vi "Read Configuration File.vi"(0 "Device Type":T1=enum."Stage", 11 "Device Function":T2=enum."Secondary", 13 "Config File Path":path) -> (2 "Configuration Name":string, 4 "Unique Notifier Name":string, 8 "Device Ports/IDs/Channels":string[](array[string]), 15 "Device Engine Path":path)   [LabVIEW 2016]
uses:
  Hardware Configuration Controls/Device Function.ctl
  Hardware Configuration Controls/Device Type.ctl
panel:
  out "File Lines":string[](array[string])
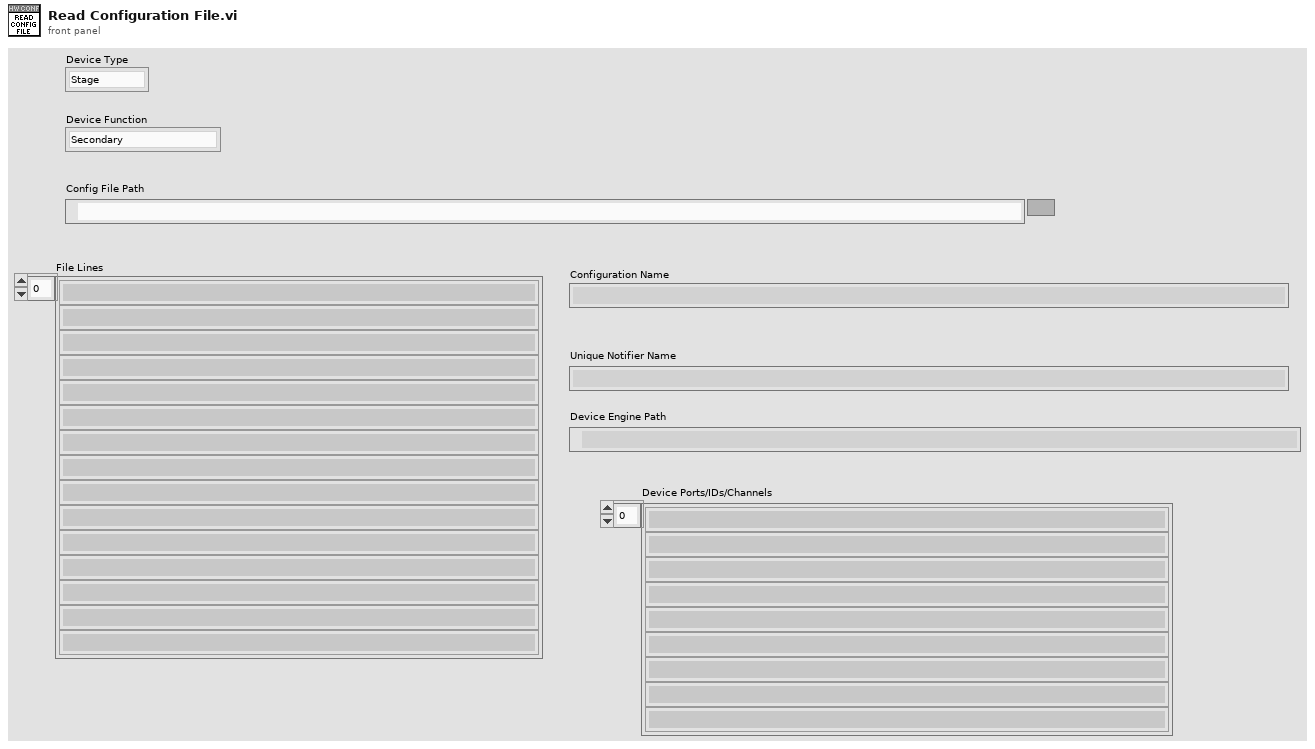
[diagram p1: front panel]
types:
  T1 = typedef "Device Type.ctl" = enum16{"AOTF", "Camera", "Deformable Mirror", "Laser", "Shutter", "Stage", "Waveform", "Email"}
  T2 = typedef "Device Function.ctl" = enum16{"Primary", "Secondary", "Overview", "Wide Field Drift Correction", "642 nm Excitation", "560 nm Excitation", "546 nm Excitation", "488 nm Excitation", "405 nm Excitation", "Objective Drift Correction", "Objective XY", "Objective Z", "Sample XY", "Sample Coarse Z", "Sample Z", "4Pi Lower", "4Pi Upper", "Adj Cavity", "Line Scanning", "Alert"}
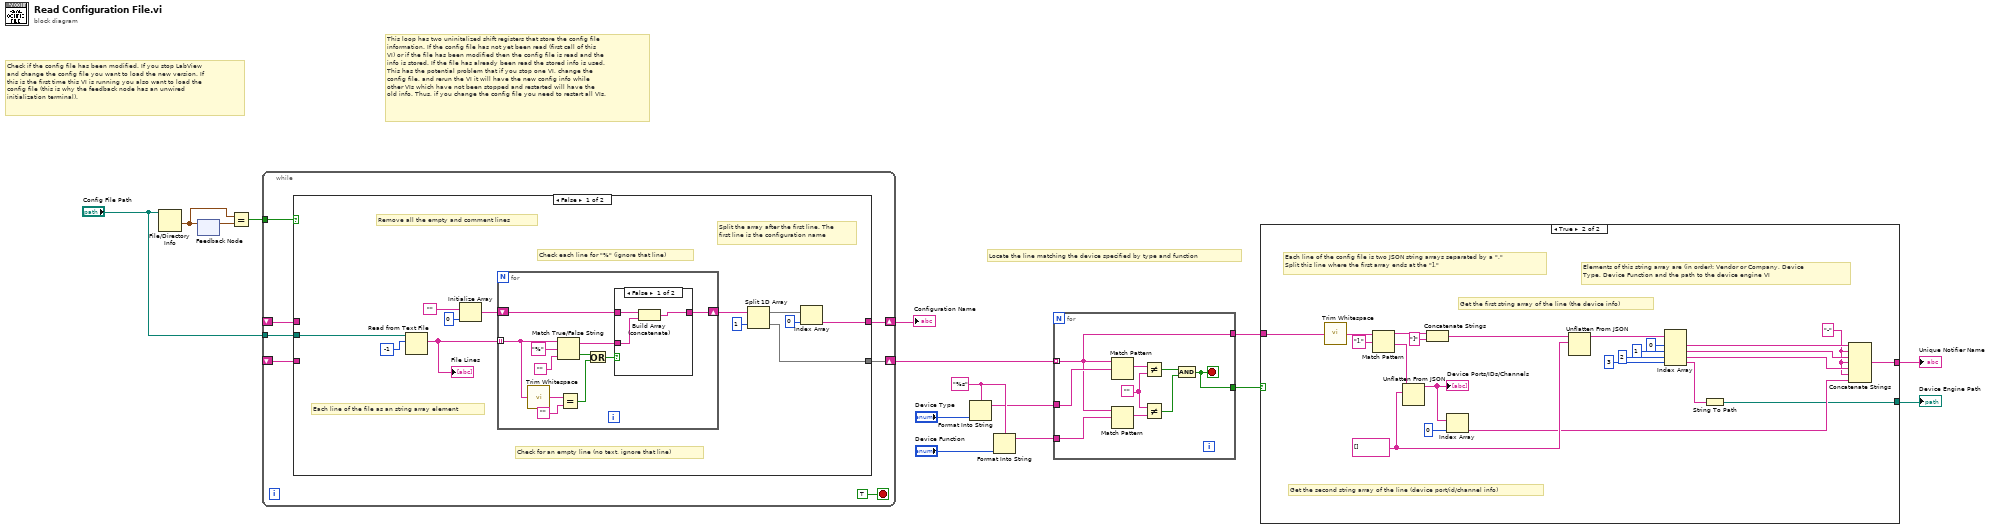
[diagram p0: block diagram]
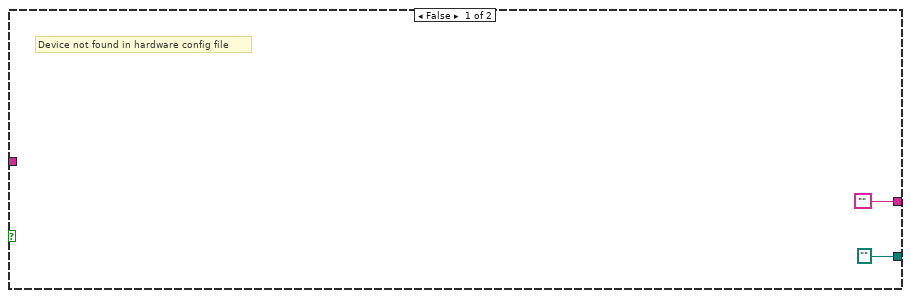
[diagram p2: hidden frame]
diagram:
  w8 = "%s" ("format string")
  # "Locate the line matching the device specified by type and function"
  # "This loop has two uninitalized shift registers that store the config file\ninformation. If the config file has not yet been read (first call of this\nVI) or if the file has been modified then the config file is read and the\ninfo is stored. If the file has already been read the stored info is used.\nThis has the potential problem that if you stop one VI, change the\nconfig file, and rerun the VI it will have the new config info while\nother VIs which have not been stopped and restarted will have the\nold info. Thus, if you change the config file you need to restart all VIs."
  # "Check if the config file has been modified. If you stop LabView\nand change the config file you want to load the new version. If\nthis is the first time this VI is running you also want to load the\nconfig file (this is why the feedback node has an unwired\ninitialization terminal)."
  n1 = File/Directory Info(path="Config File Path") -> (last mod=w13:timestamp)  [unwired: 1 in, 6 out]
  n2 = feedback-in #1(w13) -> ()
  n3 = feedback #1() -> (w14:timestamp)  [unwired: 1 in]
  n4 = Equal?(x=w13, y=w14) -> (x = y?=w12:bool)
  n5 = while {
    shift-right: [w21] -> w3
    shift-left: _ -> [w18]
    shift-right: [w22] -> w15
    shift-left: _ -> [w19]
    tunnel: w12 -> [w17]
    tunnel: "Config File Path" -> [w16]
    stop <- TRUE stop-if-true
    n6 = case shown="False" w17 {
      tunnel: [w25 w51] -> w22
      tunnel: [w24 w50] -> w21
      tunnel: w19 -> [_ w51]
      tunnel: w18 -> [_ w50]
      tunnel: w16 -> [w23 _]
      frame False {
        # "Split the array after the first line. The\nfirst line is the configuration name"
        # "Remove all the empty and comment lines"
        # "Each line of the file as an string array element"
        # "Check for an empty line (no text, ignore that line)"
        # "Check each line for \"%\" (ignore that line)"
        n7 = Read from Text File(file (use dialog)=w23, count=-1) -> (text=w33:string[])  [unwired: 2 in, 3 out]
        "File Lines" <- w33
        n8 = Initialize Array("", 0 ("dimension size")) -> (w30:string[])
        n9 = for {
          tunnel: w33 -> [w40] mode=indexing
          shift-right: [w42] -> w29
          shift-left: w30 -> [w43]
          n10 = call <vilib>:"Trim Whitespace.vi"("string"=w40) -> ("trimmed string"=w39:string)  [unwired: 1 in]
          n11 = Match True/False String(2:"", 3:"%" ("true string"), 4:w40) -> (0:w37:bool, 1:w44:string)
          n12 = Equal?(x=w39, y="") -> (x = y?=w36:bool)
          n13 = Or(x=w37, y=w36) -> (x .or. y?=w35:bool)
          n14 = case shown="False" w35 {
            tunnel: w44 -> [w46 _]
            tunnel: w43 -> [w48 w49]
            tunnel: [w47 w49] -> w42
            frame False {
              n15 = Build Array (concatenate)(w48, w46) -> (w47:string[])
            }
            frame True {
            }
          }
        }
        n16 = Split 1D Array(array=w29, index=1) -> (first subarray=w27:string[], second subarray=w24:string[])
        n17 = Index Array(array=w27, index=0) -> (element=w25:string)
      }
      frame True {
      }
    }
  }
  "Configuration Name" <- w15
  n18 = Format Into String(format string=w8, "Device Type") -> (resulting string=w6:string)  [unwired: 2 in, 1 out]
  n19 = Format Into String(format string=w8, "Device Function") -> (resulting string=w7:string)  [unwired: 2 in, 1 out]
  n20 = for {
    tunnel: w3 -> [w53] mode=indexing
    tunnel: w7 -> [w57]
    tunnel: w6 -> [w56]
    tunnel: [w53] -> w4
    tunnel: [w52] -> w2
    stop <- w52 stop-if-true
    w59 = ""
    n21 = Match Pattern(string=w53, regular expression=w56) -> (match substring=w60:string)  [unwired: 1 in, 3 out]
    n22 = Match Pattern(string=w53, regular expression=w57) -> (match substring=w58:string)  [unwired: 1 in, 3 out]
    n23 = Not Equal?(x=w60, y=w59) -> (x != y?=w55:bool)
    n24 = Not Equal?(x=w59, y=w58) -> (x != y?=w54:bool)
    n25 = And(x=w55, y=w54) -> (x .and. y?=w52:bool)
  }
  n26 = case shown="True" w2 {
    tunnel: ["" w65] -> w5
    tunnel: w4 -> [_ w64]
    tunnel: [path "" w63] -> w1
    frame False {
      # "Device not found in hardware config file"
    }
    frame True {
      w66 = "-"
      w79 = string[] []
      # "Elements of this string array are (in order): Vendor or Company, Device\nType, Device Function and the path to the device engine VI"
      # "Each line of the config file is two JSON string arrays separated by a \",\"\nSplit this line where the first array ends at the \"],\""
      # "Get the second string array of the line (device port/id/channel info)"
      # "Get the first string array of the line (the device info)"
      n27 = call <vilib>:"Trim Whitespace.vi"("string"=w64) -> ("trimmed string"=w84:string)  [unwired: 1 in]
      n28 = Match Pattern(string=w84, regular expression="],") -> (before substring=w83:string, after substring=w80:string)  [unwired: 1 in, 2 out]
      n29 = Unflatten From JSON(JSON string=w80, type and defaults=w79) -> (value=w78:string[])  [unwired: 5 in, 1 out]
      "Device Ports/IDs/Channels" <- w78
      n30 = Concatenate Strings(w83, "]" ("string")) -> (w81:string)
      n31 = Index Array(array=w78, index=0) -> (element=w67:string)
      n32 = Unflatten From JSON(JSON string=w81, type and defaults=w79) -> (value=w76:string[])  [unwired: 5 in, 1 out]
      n33 = Index Array(array=w76, index #1=0 ("index"), index #2=1 ("index"), index #3=2 ("index"), index #4=3 ("index")) -> (element #1=w70:string, element #2=w69:string, element #3=w68:string, element #4=w71:string)
      n34 = String To Path(string=w71) -> (path=w63:path)
      n35 = Concatenate Strings(w70, w66, w69, w66, w68, w66, w67) -> (w65:string)
    }
  }
  "Unique Notifier Name" <- w5
  "Device Engine Path" <- w1
